vi "Untitled 1.vi"() -> ()   [LabVIEW 2018, in "ScopePlugins.lvlib" / "NIScope.lvclass"]
uses:
  NIScope.lvclass
  C:/Users/ico/Documents/Projects/NistPluggableModules/Scope/ScopePlugins/ScopePluginBaseClass/ScopePluginsBase.lvclass
  ConnectionArray.ctl
  ScopePluginBaseClass/ScopePluginsBase.lvclass/ScopePluginsBase.ctl
  ScopePluginBaseClass/Accessors/Read Channels.vi
  ScopePluginBaseClass/Accessors/Write Channels.vi
  ScopePlugins.lvlib
panel:
  out "NIScope out":refnum<class "NIScope.lvclass">
  in  "NIScope in":refnum<class "NIScope.lvclass">
  out "error out":errorcluster
  in  "error in (no error)":errorcluster
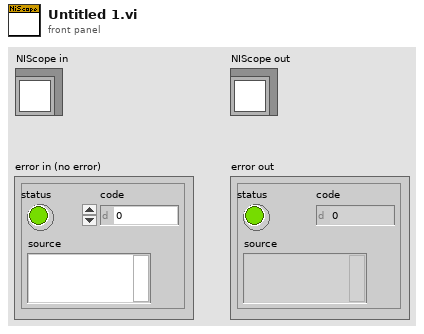
[diagram p1: front panel]
types:
  T1 = typedef "ScopePlugins.lvlib/ConnectionArray.ctl" = cluster{"Open Connection":bool, "Instrument handle":refnum<k15>}[]
  T2 = typedef "ScopePlugins.lvlib/Channels.ctl" = cluster{"Count":i32, "ChannelArray":T3[]}
  T3 = typedef "ScopePlugins.lvlib/Channel.ctl" = cluster{"Enabled":bool, "Name":string, "InputImpedance":dbl, "InputFreqMax":dbl, "ProbeAttn":dbl, "Coupling":enum16{"AC", "DC", "GND"}, "Offset":dbl, "Range":dbl, "Handle":string, "Connected":bool, "Options String ":string}
  T4 = typedef "ScopePlugins.lvlib/InitOptions.ctl" = cluster{"Reset":bool, "IdQuery":bool, "AutoConfig":bool, "Options String":string, "Synchronize":bool}
  T5 = cluster{"Open Connection (F=Open)":bool, "Instrument handle":refnum<k15>}
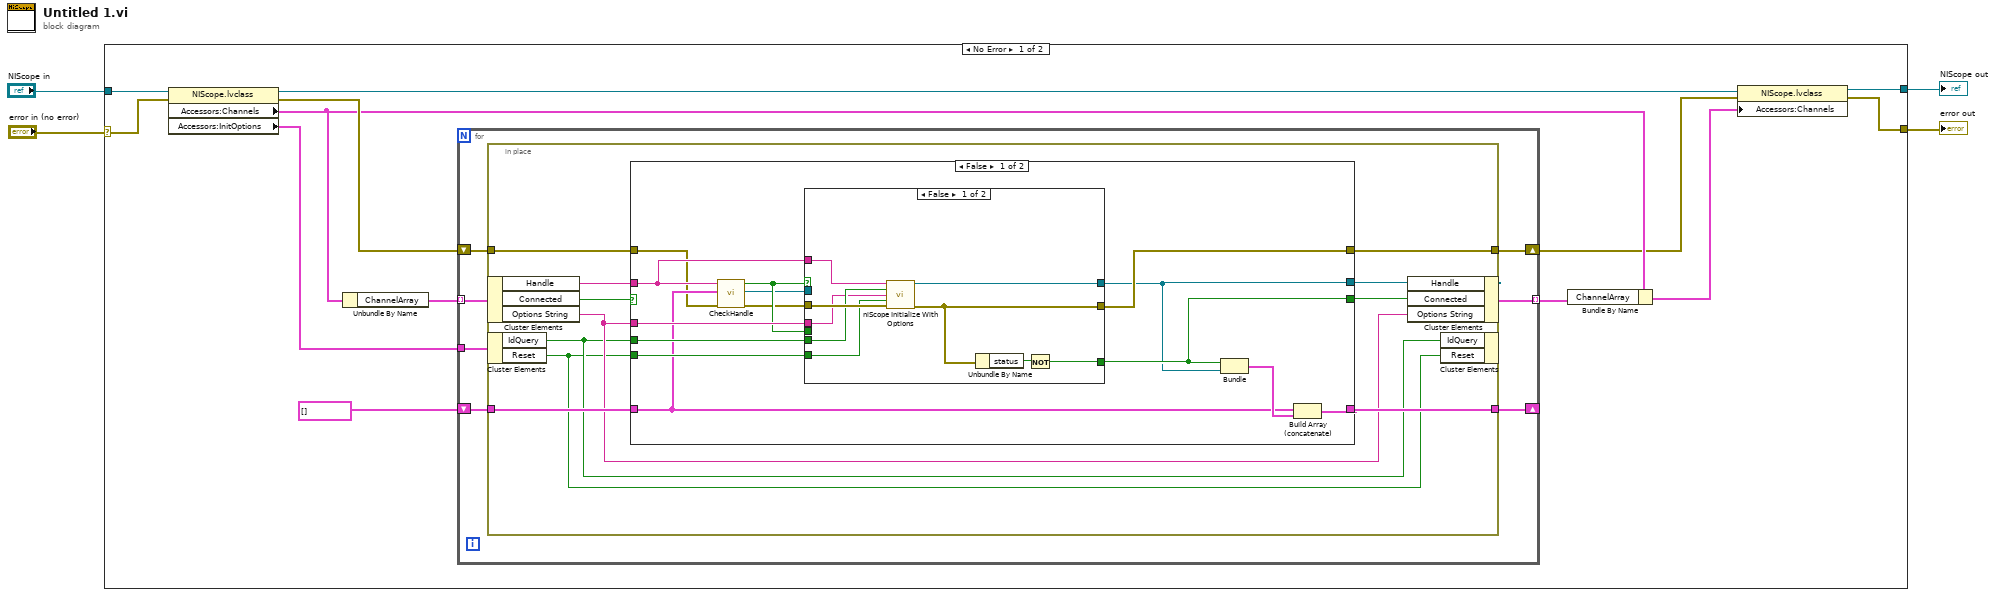
[diagram p0: block diagram]
diagram:
  n1 = case shown="No Error" "error in (no error)" {
    selector: "error in (no error)" -> [w17 w66]
    tunnel: "NIScope in" -> [w8 w67]
    tunnel: [w11 w67] -> w2
    tunnel: [w12 w66] -> w1
    frame No Error {
      n2 = property class="NIScope.lvclass"(reference=w8, error in=w17) -> (reference out=w10:refnum<class "NIScope.lvclass">, error out=w16:errorcluster, "Accessors:Channels"=w14:T2, "Accessors:InitOptions"=w6:T4)
      n3 = Unbundle By Name(w14) -> ("ChannelArray"=w5:T3[])
      n4 = for {
        tunnel: w5 -> [w24] mode=indexing
        shift-right: [w20] -> w9
        shift-left: w16 -> [w23]
        shift-right: [w21] -> _
        shift-left: T1 [] ("Connection Array") -> [w22]
        tunnel: [w19] -> w15 mode=indexing
        tunnel: w6 -> [w18]
        n5 = in-place {
          in-place-border: w23 -> [w34]
          in-place-border: w22 -> [w33]
          in-place-border: [w31] -> w21
          in-place-border: [w30] -> w20
          n6 = in-place-cluster #1(w24) -> ("Handle"=w27:string, "Connected"=w35:bool, "Options String"=w29:string)
          n7 = in-place-cluster #2(w18) -> ("IdQuery"=w26:bool, "Reset"=w25:bool)
          n8 = case shown="False" w35 {
            selector: w35 -> [_ w64]
            tunnel: w34 -> [w38 w65]
            tunnel: w27 -> [w41 w63]
            tunnel: w26 -> [w49 _]
            tunnel: w25 -> [w48 _]
            tunnel: w33 -> [w40 w62]
            tunnel: [w47 w64] -> w32
            tunnel: [w43 w63] -> w28
            tunnel: [w45 w62] -> w31
            tunnel: [w44 w65] -> w30
            tunnel: w29 -> [w42 _]
            frame False {
              n9 = call "CheckHandle.vi"("error in (no error)"=w38, "Connection Array"=w40, "Handle In"=w41) -> ("error out"=w37:errorcluster, "Instrument handle"=w36:refnum<k15>, "Open Connection (F=Open)"=w39:bool)  [unwired: 5 in, 1 out]
              n10 = case shown="False" w39 {
                tunnel: w41 -> [w58 _]
                tunnel: w37 -> [w57 w60]
                tunnel: [w52 w60] -> w44
                tunnel: [w51 w59] -> w43
                tunnel: w49 -> [w56 _]
                tunnel: w48 -> [w55 _]
                tunnel: [w53 w61] -> w47
                tunnel: w39 -> [_ w61]
                tunnel: w36 -> [_ w59]
                tunnel: w42 -> [w50 _]
                frame False {
                  n11 = call <instrlib>:"niScope Initialize With Options.vi"("resource name"=w58, "id query"=w56, "option string"=w50, "reset device"=w55, "error in"=w57) -> ("instrument handle"=w51:refnum<k15>, "error out"=w52:errorcluster)  [unwired: 9 in]
                  n12 = Unbundle By Name(w52) -> ("status"=w54:bool)
                  n13 = Not(x=w54) -> (.not. x?=w53:bool)
                }
                frame True {
                }
              }
              n14 = Bundle("Open Connection (F=Open)"=w47, "Instrument handle"=w43) -> (w46:T5)  [unwired: 1 in]
              n15 = Build Array (concatenate)(w40, w46) -> (w45:T1)
            }
            frame True {
            }
          }
          n16 = in-place-cluster #1("Handle"=w28, "Connected"=w32, "Options String"=w29) -> (w19:T3)
          n17 = in-place-cluster #2("IdQuery"=w26, "Reset"=w25) -> ()  [unwired: 1 out]
        }
      }
      n18 = Bundle By Name(cluster=w14, "ChannelArray"=w15) -> (w13:T2)
      n19 = property class="NIScope.lvclass"(reference=w10, error in=w9, "Accessors:Channels"=w13) -> (reference out=w11:refnum<class "NIScope.lvclass">, error out=w12:errorcluster)
    }
    frame Error {
    }
  }
  "error out" <- w1
  "NIScope out" <- w2
